vi "ms us ns 2 double.vi"(0 "sec":i32, 5 "ms":i32, 7 "µs":i32 min=-1000 max=1000, 9 "ns":i32 min=-1000 max=1000, 11 "ps":i32 min=-1000 max=1000) -> (8 "µs":dbl format="%#.9g")   [LabVIEW 2009, in "CS POLARIS BME DG Client.lvlib"]
uses:
  CS POLARIS BME DG Client.lvlib
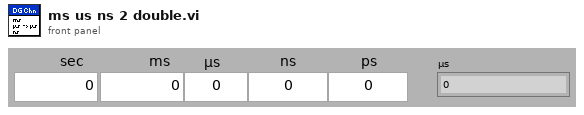
[diagram p1: front panel]
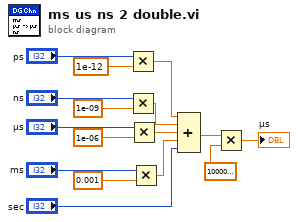
[diagram p0: block diagram]
diagram:
  n1 = Multiply(x="ps", y=1e-12) -> (x*y=w1:dbl)
  n2 = Multiply(x="ns", y=1e-09) -> (x*y=w4:dbl)
  n3 = Multiply(x="µs", y=1e-06) -> (x*y=w11:dbl)
  n4 = Multiply(x="ms", y=0.001) -> (x*y=w6:dbl)
  n5 = Compound Arithmetic op=ADD(w1, w4, w11, w6, "sec") -> (w10:dbl)
  n6 = Multiply(x=w10, y=1000000.0) -> (x*y=→"µs":dbl)
